vi "PH_ImageOperator.CreateTrace.vi"(1 "Calibrate":bool, 2 "Calibration Factor":dbl, 3 "Offset":sgl, 4 "Trace":sgl[](array[numeric])) -> (16 "calibrated":bool, 17 "Trace Output":cluster{"Index":sgl[], "Trace":sgl[]})   [LabVIEW 2014, in "PH_ImageOperator.lvlib"]
doc: "This VI creates the Trace the Gaussian function is fitted to."
uses:
  PH_ImageOperator.lvlib
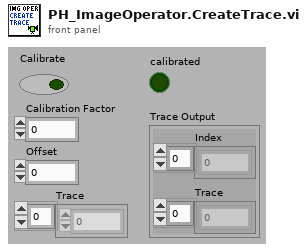
[diagram p1: front panel]
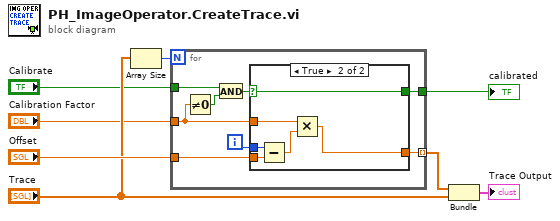
[diagram p0: block diagram]
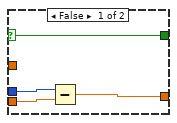
[diagram p2: hidden frame]
diagram:
  n1 = Array Size(array="Trace") -> (size(s)=w5:i32)
  n2 = for {
    N: w5 -> [_]
    tunnel: "Offset" -> [w16]
    tunnel: [w15] -> w7 mode=indexing
    tunnel: "Calibrate" -> [w11]
    tunnel: "Calibration Factor" -> [w13]
    tunnel: [w9] -> w1
    i -> [w14]
    n3 = Not Equal To 0?(x=w13) -> (x != 0?=w12:bool)
    n4 = And(x=w11, y=w12) -> (x .and. y?=w10:bool)
    n5 = case shown="True" w10 {
      selector: w10 -> [w17 w21]
      tunnel: w16 -> [w20 w26]
      tunnel: [w19 w22] -> w15
      tunnel: w14 -> [w18 w25]
      tunnel: w13 -> [_ w23]
      tunnel: [w17 w21] -> w9
      frame False {
        n6 = Subtract(x=w18, y=w20) -> (x-y=w19:sgl)
      }
      frame True {
        n7 = Subtract(x=w25, y=w26) -> (x-y=w24:sgl)
        n8 = Multiply(x=w23, y=w24) -> (x*y=w22:dbl)
      }
    }
  }
  "calibrated" <- w1
  n9 = Bundle(w7, "Trace"="Trace") -> (→"Trace Output":cluster{dbl[], "Trace":sgl[]})  [unwired: 1 in]
